vi "MoveWindow.vi"(4 "error in (no error)":errorcluster, 7 "hWnd (NULL)":T1) -> (0 "error out":errorcluster, 3 "dup hWnd":T1)   [LabVIEW 2011]
doc: "MoveWindow\nThe MoveWindow function changes the position and dimensions of the specified window. For a top-level window, the position and dimensions are relative to the upper-left corner of the screen. For a child window, they are relative to the upper-left corner of the parent window's client area. \n\nBOOL MoveWindow(\n HWND hWnd, // handle to window\n int X, // horizontal position\n int Y, // vertical position\n int nWidth, // width\n int nHeight, // height\n BOOL bRepaint // repaint flag\n);\n \nParameters\nhWnd \nHandle to the window. \nX \nSpecifies the new position of the left side of the window. \nY \nSpecifies the new position of the top of the window. \nnWidth \nSpecifies the new width of the window. \nnHeight \nSpecifies the new height of the window. \nbRepaint \nSpecifies whether the window is to be repainted. If this parameter is TRUE, the window receives aWM_PAINT message. If the parameter is FALSE, no repainting of any kind occurs. This applies to the client area, the nonclient area (including the title bar and scroll bars), and any part of the parent window uncovered as a result of moving a child window. If this parameter is FALSE, the application must explicitly invalidate or redraw any parts of the window and parent window that need redrawing. \nReturn Values\nIf the function succeeds, the return value is nonzero.\n\nIf the function fails, the return value is zero. To get extended error information, callGetLastError.\n\nRemarks\nIf the bRepaint parameter is TRUE, the system sends the WM_PAINT message to the window procedure immediately after moving the window (that is, the MoveWindow function calls the UpdateWindow function). If bRepaint is FALSE, the system places the WM_PAINT message in the message queue associated with the window. The message loop dispatches the WM_PAINT message only after dispatching all other messages in the queue. \n\nMoveWindow sends WM_WINDOWPOSCHANGING, WM_WINDOWPOSCHANGED, WM_MOVE, WM_SIZE, and WM_NCCALCSIZE messages to the window."
uses:
  hWnd.ctl
  user32.dll
panel:
  in  "Repaint? (T)":bool=TRUE
  in  "Metrics (0,0,0,0)":cluster{"X":i32, "Y":i32, "cx":i32, "cy":i32}
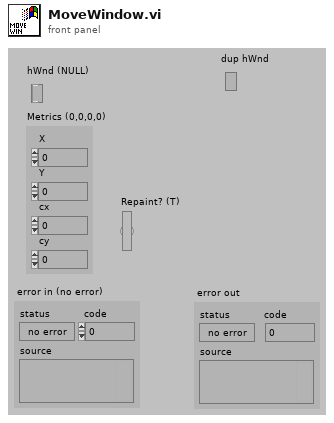
[diagram p1: front panel]
types:
  T1 = typedef "hWnd.ctl" = refnum<k1>
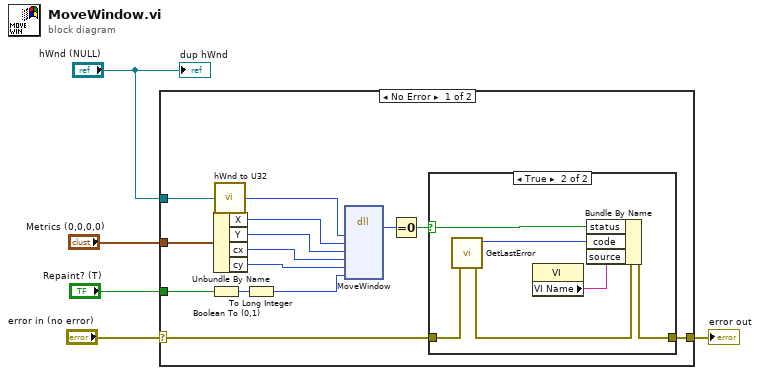
[diagram p0: block diagram]
diagram:
  n1 = case shown="No Error" "error in (no error)" {
    selector: "error in (no error)" -> [w13 w27]
    tunnel: [w17 w27] -> w4
    tunnel: "Metrics (0,0,0,0)" -> [w10 _]
    tunnel: "hWnd (NULL)" -> [w12 _]
    tunnel: "Repaint? (T)" -> [w14 _]
    frame No Error {
      n2 = Boolean To (0,1)(Boolean=w14) -> (0, 1=w19:i16)
      n3 = Unbundle By Name(w10) -> ("X"=w9:i32, "Y"=w8:i32, "cx"=w7:i32, "cy"=w6:i32)
      n4 = call "hWnd to U32.vi"("hWnd"=w12) -> ("hWnd"=w11:u32)  [unwired: 4 out]
      n5 = To Long Integer(number=w19) -> (32bit integer=w15:i32)
      n6 = dll-call lib="User32.dll" fn="MoveWindow"("hWnd"=w11, "X"=w9, "Y"=w8, "cx"=w7, "cy"=w6, "repaint"=w15) -> ("error"=w18:i32)  [unwired: 9 in, 2 out]
      n7 = Equal To 0?(x=w18) -> (x = 0?=w16:bool)
      n8 = case shown="True" w16 {
        selector: w16 -> [_ w21]
        tunnel: w13 -> [w20 w25]
        tunnel: [w20 w26] -> w17
        frame False {
        }
        frame True {
          n9 = call "GetLastError.vi"("error in (no error)"=w25) -> ("error out"=w24:errorcluster, "CODE"=w23:i32)  [unwired: 5 out]
          n10 = property class="VI"() -> ("VI Name"=w22:string)  [unwired: 2 in, 2 out]
          n11 = Bundle By Name(cluster=w24, "status"=w21, "code"=w23, "source"=w22) -> (w26:errorcluster)
        }
      }
    }
    frame Error {
    }
  }
  "error out" <- w4
  "dup hWnd" <- "hWnd (NULL)"
